vi "Esercitazione 4 - Fattoriale.vi"() -> ()   [LabVIEW 2018]
panel:
  out "Numeric 4":i32
  out "Numeric 2":i32
  in  "Numeric":i32
  in  "Numeric 3":i32
  in  "stop":bool
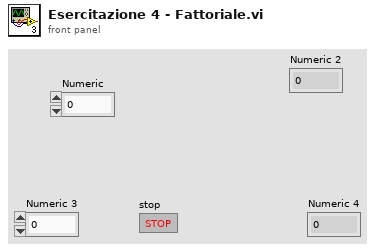
[diagram p1: front panel]
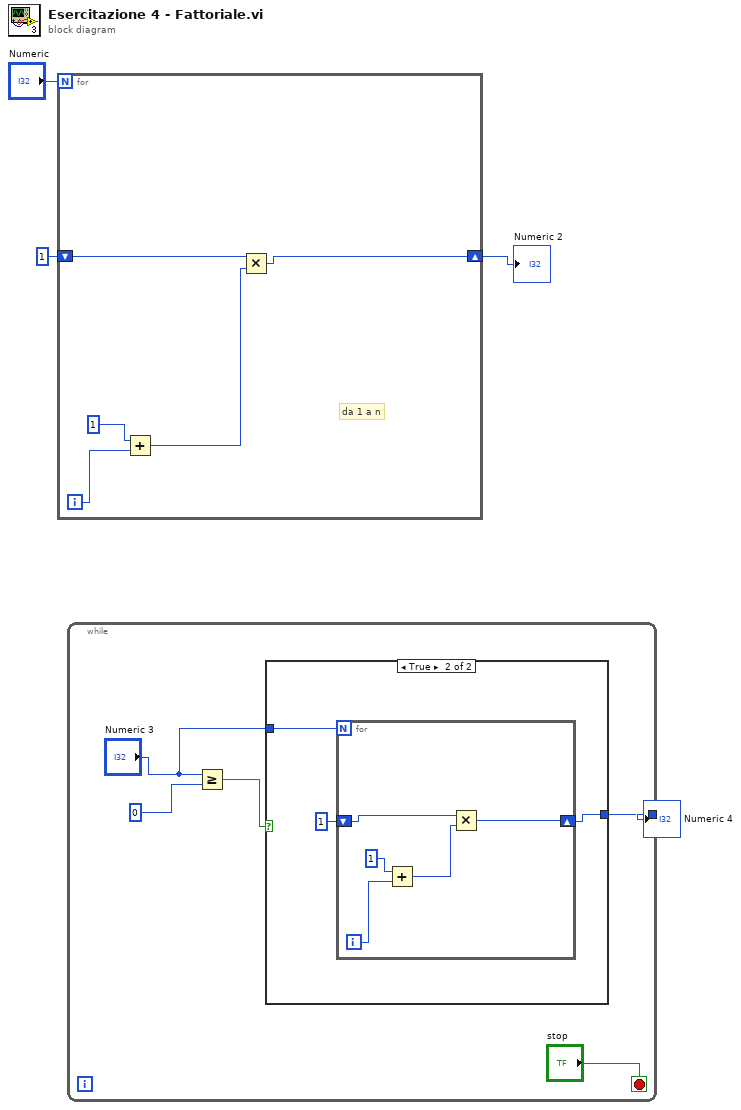
[diagram p0: block diagram]
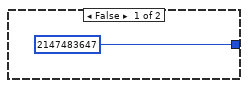
[diagram p2: hidden frame]
diagram:
  n1 = for {
    N: "Numeric" -> [_]
    shift-right: [w9] -> w3
    shift-left: 1 -> [w8]
    i -> [w7]
    # "da 1 a n"
    n2 = Add(x=1 ("y"), y=w7) -> (x+y=w5:i32)
    n3 = Multiply(x=w8, y=w5) -> (x*y=w9:i32)
  }
  "Numeric 2" <- w3
  n4 = while {
    tunnel: [w10] -> w1
    stop <- "stop" stop-if-true
    n5 = Greater Or Equal?(x="Numeric 3", y=0) -> (x >= y?=w12:bool)
    n6 = case shown="True" w12 {
      tunnel: "Numeric 3" -> [_ w18]
      tunnel: [2147483647 w16] -> w10
      frame False {
      }
      frame True {
        n7 = for {
          N: w18 -> [_]
          shift-right: [w20] -> w16
          shift-left: 1 -> [w19]
          i -> [w23]
          n8 = Add(x=1, y=w23) -> (x+y=w21:i32)
          n9 = Multiply(x=w19, y=w21) -> (x*y=w20:i32)
        }
      }
    }
  }
  "Numeric 4" <- w1
